vi "GetCodePaths.vi"(8 "stringIn":string, 11 "pythonCodes":cluster{"pythonCode":path, "Color":u32}[](array[cluster])) -> (0 "Paths out":path[](array[path]), 1 "pythonCodes out":cluster{"pythonCode":path, "Color":u32}[](array[cluster]), 3 "stringOut":string)   [LabVIEW 2022 SP3]
uses:
  <vilib>/Utility/error.llb/Trim Whitespace One-Sided.vi
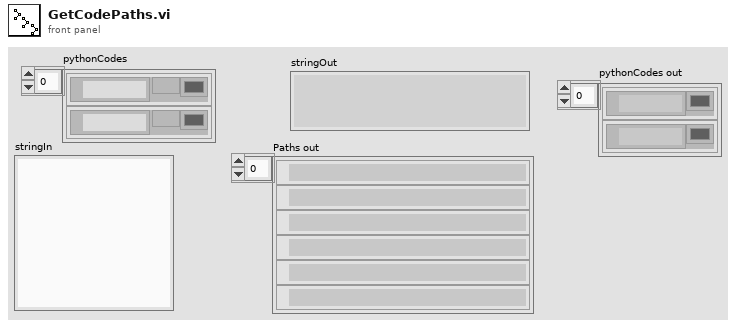
[diagram p1: front panel]
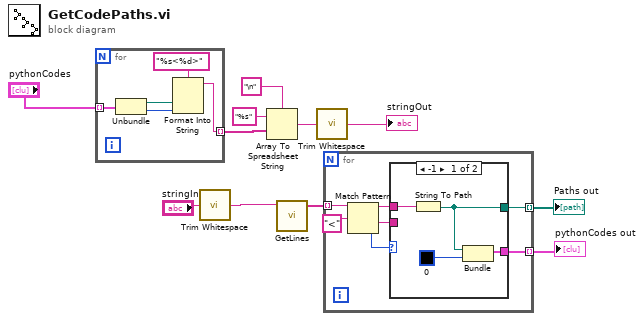
[diagram p0: block diagram]
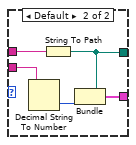
[diagram p2: hidden frame]
diagram:
  n1 = for {
    tunnel: "pythonCodes" -> [w16] mode=indexing
    tunnel: [w12] -> w4 mode=indexing
    n2 = Unbundle(w16) -> ("pythonCode"=w14:path, "Color"=w13:u32)
    n3 = Format Into String(format string="%s<%d>", w14, w13) -> (resulting string=w12:string)  [unwired: 2 in, 1 out]
  }
  n4 = call <vilib>:"Trim Whitespace.vi"("string"="stringIn") -> ("trimmed string"=w2:string)  [unwired: 1 in]
  n5 = Array To Spreadsheet String(delimiter (Tab)="\n", array=w4, 3:"%s" ("format string")) -> (spreadsheet string=w11:string)
  n6 = call "GetLines.vi"("String"=w2) -> ("Array"=w1:string[])  [unwired: 10 in]
  n7 = call <vilib>:"Trim Whitespace.vi"("string"=w11) -> ("trimmed string"=→"stringOut":string)  [unwired: 1 in]
  n8 = for {
    tunnel: w1 -> [w21] mode=indexing
    tunnel: [w22] -> w7 mode=indexing
    tunnel: [w23] -> w3 mode=indexing
    n9 = Match Pattern(string=w21, regular expression="<" ("format string")) -> (before substring=w19:string, after substring=w18:string, offset past match=w17:i32)  [unwired: 1 in, 1 out]
    n10 = case shown="-1" w17 {
      tunnel: [w24 w32] -> w23
      tunnel: [w26 w31] -> w22
      tunnel: w19 -> [w27 w30]
      tunnel: w18 -> [_ w29]
      frame -1 {
        n11 = String To Path(string=w27) -> (path=w26:path)
        n12 = Bundle(w26, u32 0) -> (w24:cluster{path, u32})  [unwired: 1 in]
      }
      frame Default {
        n13 = Decimal String To Number(string=w29) -> (number=w28:i32)  [unwired: 2 in, 1 out]
        n14 = String To Path(string=w30) -> (path=w31:path)
        n15 = Bundle(w31, w28) -> (w32:cluster{path, i32})  [unwired: 1 in]
      }
    }
  }
  "Paths out" <- w7
  "pythonCodes out" <- w3
